vi "Source Current.vi"(8 "error in (no error)":errorcluster, 9 "Pin":string, 10 "Current level":dbl caption="current level" format="%_6p", 11 "Semiconductor Module Context":T1) -> (0 "error out":errorcluster, 1 "current measurements":dbl[](array[numeric]), 2 "voltage measurements":dbl[](array[numeric]), 3 "Semiconductor Module Context Out":T1)   [LabVIEW 2013]
uses:
  <vilib>/NI_TestStand_SemiconductorModule/NI_TestStand_Semiconductor_Module.lvlibp/PinMap/General/SemiconductorModuleContext.ctl
  <instrlib>/niDCPower/nidcpower.llb/niDCPower Wait For Event - Event.ctl
  <vilib>/NI_TestStand_SemiconductorModule/NI_TestStand_Semiconductor_Module.lvlibp/PinMap/DC Power/PinToNIDCPowerSession.vi
  <vilib>/NI_TestStand_SemiconductorModule/NI_TestStand_Semiconductor_Module.lvlibp
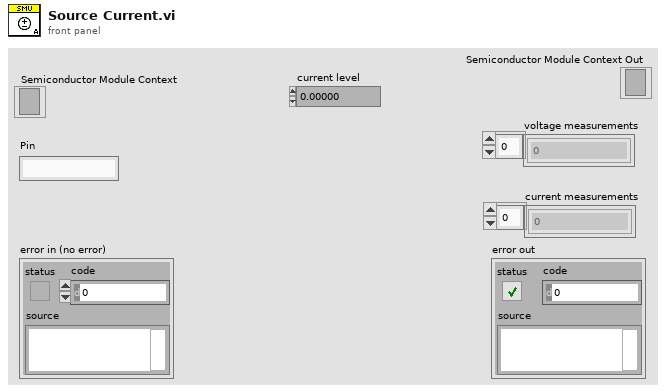
[diagram p1: front panel]
types:
  T1 = typedef "NI_TestStand_Semiconductor_Module.lvlibp/SemiconductorModuleContext.ctl" = refnum<k7>
  T2 = typedef "niDCPower Wait For Event - Event.ctl" = i32
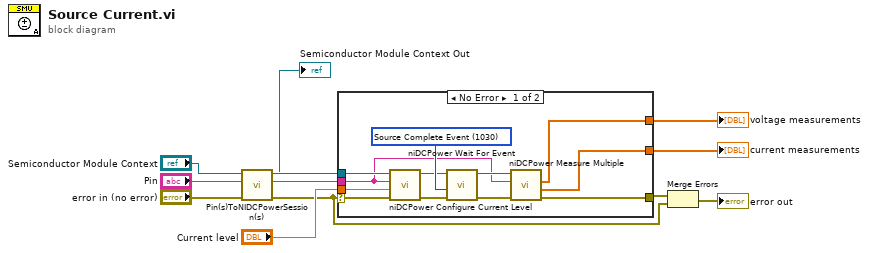
[diagram p0: block diagram]
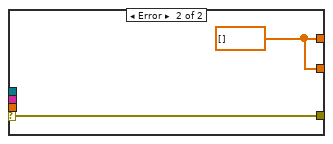
[diagram p2: hidden frame]
diagram:
  n1 = call-poly <vilib>:"Pin(s)ToNIDCPowerSession(s).vi"("error in (no error)"="error in (no error)", "Pin"="Pin", "Semiconductor Module Context"="Semiconductor Module Context") -> ("error out"=w5:errorcluster, "Instrument Session"=w10:refnum<k15>, "Channel List"=w9:string, "Semiconductor Module Context Out"=→"Semiconductor Module Context Out":T1)  [unwired: 4 in, 1 out]
  n2 = case shown="No Error" w5 {
    selector: w5 -> [w18 w26]
    tunnel: [w19 w26] -> w4
    tunnel: w10 -> [w15 _]
    tunnel: w9 -> [w14 _]
    tunnel: "Current level" -> [w13 _]
    tunnel: [w21 w25] -> w3
    tunnel: [w20 w25] -> w6
    frame No Error {
      w24 = T2 1030 items=["Source Complete Event"=1030, "Measure Complete Event"=1031, "Sequence Iteration Complete Event"=1032, "Sequence Engine Done Event"=1033, "Pulse Complete Event"=1051, "Ready For Pulse Trigger Event"=1052] ("event")
      n3 = call <instrlib>:"niDCPower Configure Current Level.vi"("error in (no error)"=w18, "current level"=w13, "channel name"=w14, "instrument handle"=w15) -> ("error out"=w17:errorcluster, "instrument handle out"=w16:refnum<k15>)  [unwired: 6 in]
      n4 = call <instrlib>:"niDCPower Wait For Event.vi"("error in (no error)"=w17, "event"=w24, "instrument handle"=w16) -> ("error out"=w23:errorcluster, "instrument handle out"=w22:refnum<k15>)  [unwired: 7 in]
      n5 = call <instrlib>:"niDCPower Measure Multiple.vi"("error in (no error)"=w23, "channel name"=w14, "instrument handle"=w22) -> ("error out"=w19:errorcluster, "current measurements"=w20:dbl[], "voltage measurements"=w21:dbl[])  [unwired: 5 in, 1 out]
    }
    frame Error {
      w25 = dbl[] [] ("voltage measurements")
    }
  }
  "voltage measurements" <- w3
  "current measurements" <- w6
  n6 = Merge Errors(w4, w5) -> (→"error out":errorcluster)
